vi "Read Item.vi"(6 "itemName":string, 8 "error in (no error)":errorcluster, 11 ".NET Refnum in":refnum<k24>) -> (0 "error out":errorcluster, 1 "variant":variant, 2 "Value (SGL/DBL only!)":dbl, 3 ".NET Refnum out":refnum<k24>, 4 "type":T1, 5 "ItemName":string, 7 "Name":string)   [LabVIEW 2024, in "LV_OPC_NET.lvlib"]
uses:
  LV_OPC_NET.lvlib
  <vilib>/Utility/Data Type/Type Definitions/Data Type.ctl
  C:/Users/Andrey/Desktop/LV_OPC-Client-x64/LV_OPC_Test/OPC.NET/OpcNetApi.dll
  OpcNetApi.dll
  System.Xml
  <vilib>/Utility/Data Type/NI_Data Type.lvlib
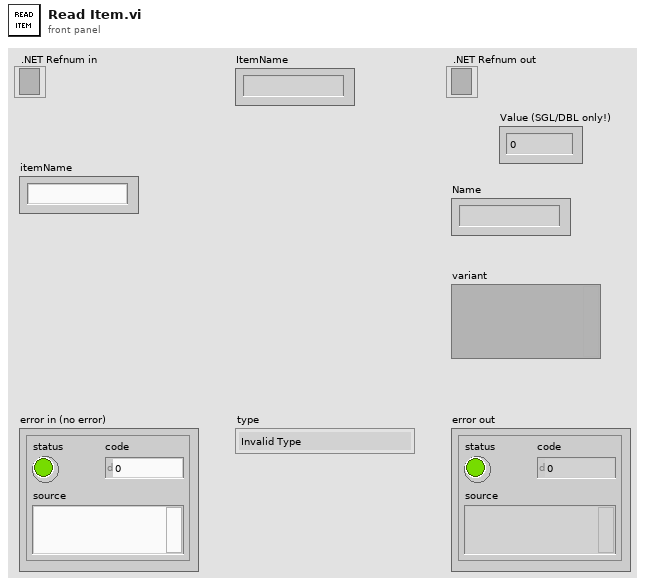
[diagram p1: front panel]
types:
  T1 = typedef "NI_Data Type.lvlib/Data Type.ctl" = enum8{"Invalid Type", "Void", "I8", "I16", "I32", "I64", "U8", "U16", "U32", "U64", "Single Float", "Double Float", "Extended Float", "Single Complex", "Double Complex", "Extended Complex", "Enum U8", "Enum U16", "Enum U32", "Enum U64", "Single Float With Unit", "Double Float With Unit", "Extended Float With Unit", "Single Complex with Unit", "Double Complex with Unit", "Extended Complex with Unit", "Boolean", "String", "Path", "Picture", "Tag", "Array", "Cluster", "Variant", "LV Variant", "Waveform", "Timestamp", "Digital Waveform", "Digital Data", "ExpressData", "Refnum", "External Data", "VI", "Poly VI", "LabVIEW Class Instance", "Fixed Point", "Set Collection", "Map Collection"}
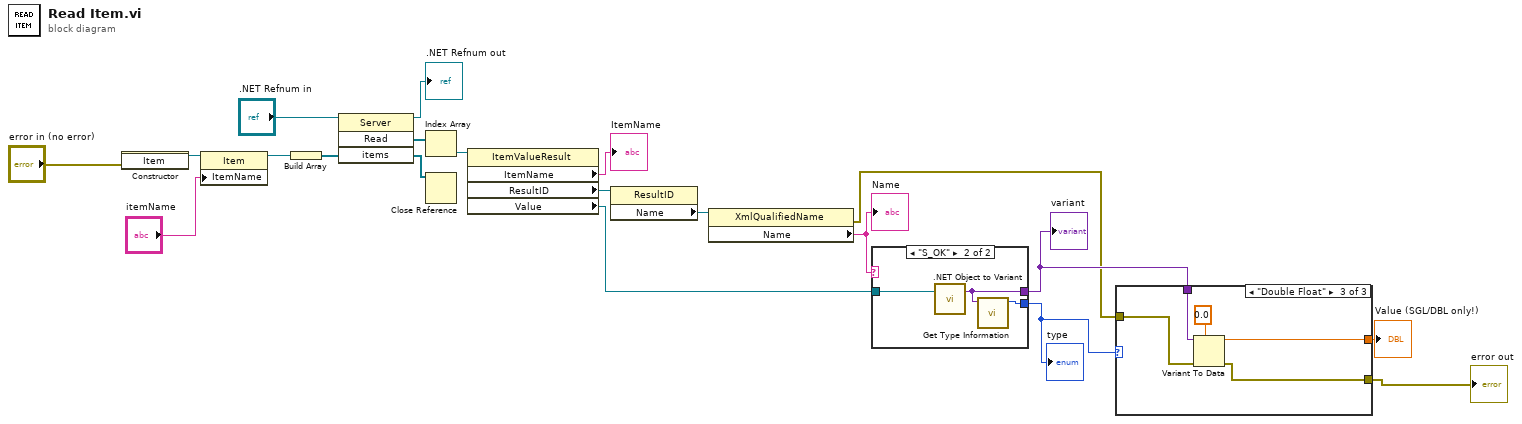
[diagram p0: block diagram]
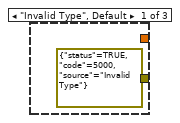
[diagram p2: hidden frame]
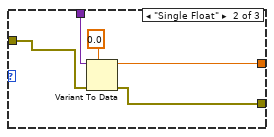
[diagram p3: hidden frame]
diagram:
  n1 = constructor class="Item"(error in="error in (no error)") -> (reference out=w8:refnum<k24>)  [unwired: 2 in, 2 out]
  n2 = property class="Item"(reference=w8, "ItemName"="itemName") -> (reference out=w9:refnum<k24>)  [unwired: 1 in, 1 out]
  n3 = Build Array(w9) -> (w10:refnum<k24>[])
  n4 = invoke class="Server" method="Read"(reference=".NET Refnum in", "items"=w10) -> (reference out=→".NET Refnum out":refnum<k24>, "Read"=w16:refnum<k24>[], "items"=w15:refnum<k24>[])  [unwired: 2 in, 1 out]
  n5 = Index Array(array=w16) -> (element=w12:refnum<k24>)  [unwired: 1 in]
  n6 = Close Reference(reference=w15) -> ()  [unwired: 1 in, 1 out]
  n7 = property class="ItemValueResult"(reference=w12) -> ("ItemName"=→"ItemName":string, "ResultID"=w18:refnum<k24>, "Value"=w14:refnum<k24>)  [unwired: 1 in, 2 out]
  n8 = property class="ResultID"(reference=w18) -> ("Name"=w17:refnum<k24>)  [unwired: 1 in, 2 out]
  n9 = property class="XmlQualifiedName"(reference=w17) -> (error out=w2:errorcluster, "Name"=w19:string)  [unwired: 1 in, 1 out]
  "Name" <- w19
  n10 = case shown="\"S_OK\"" w19 {
    tunnel: w14 -> [_ w23]
    tunnel: [_ w22] -> w5
    tunnel: [_ w21] -> w4
    frame Default {
    }
    frame "S_OK" {
      n11 = call <vilib>:".NET Object to Variant.vi"(".NET object"=w23) -> ("variant"=w21:variant)  [unwired: 1 in, 1 out]
      n12 = call <vilib>:"Get Type Information.vi"("variant"=w21) -> ("type"=w22:T1)  [unwired: 6 in, 4 out]
    }
  }
  "variant" <- w4
  "type" <- w5
  n13 = case shown="\"Double Float\"" w5 {
    tunnel: w4 -> [_ w29 w34]
    tunnel: [_ w27 w32] -> w3
    tunnel: w2 -> [_ w26 w31]
    tunnel: [errorcluster {"status"=TRUE, "code"=5000, "source"="Invalid Type"} ("error out") w25 w30] -> w1
    frame "Invalid Type", Default {
    }
    frame "Single Float" {
      n14 = Variant To Data(error in=w26, type=sgl 0.0, Variant=w29) -> (data=w27:sgl, error out=w25:errorcluster)
    }
    frame "Double Float" {
      n15 = Variant To Data(error in=w31, type=0.0, Variant=w34) -> (data=w32:dbl, error out=w30:errorcluster)
    }
  }
  "error out" <- w1
  "Value (SGL/DBL only!)" <- w3
